vi "Home Caller.vi"   [LabVIEW 2015, in "Endigit.lvlib"]
uses:
  Endigit.lvlib
  <vilib>/Utility/miscctls.llb/LVPointTypeDef.ctl
panel:
  # "NOTICE - YOU MUST NOT REMOVE THIS NOTICE. PER THE FOLLOWING LICENSE, YOU MAY REPRODUCE THIS SOFTWARE PROVIDED YOU FOLLOW THE TERMS\nOF THE LICENSE.\n\n---BEGIN BSD LICENSE (http://opensource.org/licenses/BSD-2-Clause)---\nCopyright (c) 2015, Endigit, Inc. <robert@endigit.com>\nAll rights reserved.\n\nRedistribution and use in source and binary forms, with or without modification, are permitted provided that the following conditions are met:\n\n1. Redistributions of source code must retain the above copyright notice, this list of conditions and the following disclaimer.\n\n2. Redistributions in binary form must reproduce the above copyright notice, this list of conditions and the following disclaimer in the documentation and/or other \nmaterials provided with the distribution.\n\nTHIS SOFTWARE IS PROVIDED BY THE COPYRIGHT HOLDERS AND CONTRIBUTORS \"AS IS\" AND ANY EXPRESS OR IMPLIED WARRANTIES, INCLUDING, BUT NOT \nLIMITED TO, THE IMPLIED WARRANTIES OF MERCHANTABILITY AND FITNESS FOR A PARTICULAR PURPOSE ARE DISCLAIMED. IN NO EVENT SHALL THE COPYRIGHT \nHOLDER OR CONTRIBUTORS BE LIABLE FOR ANY DIRECT, INDIRECT, INCIDENTAL, SPECIAL, EXEMPLARY, OR CONSEQUENTIAL DAMAGES (INCLUDING, BUT NOT \nLIMITED TO, PROCUREMENT OF SUBSTITUTE GOODS OR SERVICES; LOSS OF USE, DATA, OR PROFITS; OR BUSINESS INTERRUPTION) HOWEVER CAUSED AND ON \nANY THEORY OF LIABILITY, WHETHER IN CONTRACT, STRICT LIABILITY, OR TORT (INCLUDING NEGLIGENCE OR OTHERWISE) ARISING IN ANY WAY OUT OF THE USE \nOF THIS SOFTWARE, EVEN IF ADVISED OF THE POSSIBILITY OF SUCH DAMAGE.\n---END BSD LICENSE---"
types:
  T1 = typedef "LVPointTypeDef.ctl" = cluster{"Horizontal":i16, "Vertical":i16}
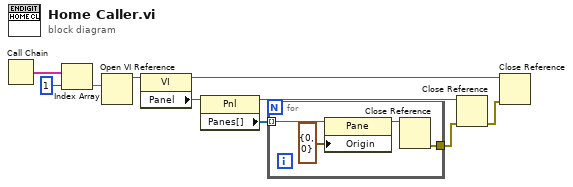
[diagram p0: block diagram]
diagram:
  n1 = Call Chain() -> (call chain=w7:string[])
  n2 = Index Array(array=w7, index=1) -> (element=w6:string)
  n3 = Open VI Reference(vi path=w6) -> (vi reference=w8:refnum<vi>)  [unwired: 5 in, 1 out]
  n4 = property class="VI"(reference=w8) -> (reference out=w2:refnum<vi>, "Panel"=w10:refnum<vi>)  [unwired: 1 in, 1 out]
  n5 = property class="Pnl"(reference=w10) -> (reference out=w4:refnum<vi>, "Panes[]"=w9:refnum<vi>[])  [unwired: 1 in, 1 out]
  n6 = for {
    tunnel: w9 -> [w14] mode=indexing
    tunnel: [w11] -> w3
    n7 = property class="Pane"(reference=w14, "Origin"=T1 {"Horizontal"=0, "Vertical"=0} ("Horizontal Scrollbar Visibility")) -> (reference out=w12:refnum<vi>)  [unwired: 1 in, 1 out]
    n8 = Close Reference(reference=w12) -> (error out=w11:errorcluster)  [unwired: 1 in]
  }
  n9 = Close Reference(reference=w4, error in (no error)=w3) -> (error out=w1:errorcluster)
  n10 = Close Reference(reference=w2, error in (no error)=w1) -> ()  [unwired: 1 out]
